vi "Value Change.vi"(8 "error in (no error)":errorcluster, 9 "NewVal":i32, 10 "Debugger":refnum<class "Debug Process.lvclass">, 11 "List Box View Model In":refnum<class "Multicolumn List Box View Model.lvclass">) -> (0 "error out":errorcluster, 3 "List Box View Model Out":refnum<class "Multicolumn List Box View Model.lvclass">)   [LabVIEW 2020, in "Multicolumn List Box View Model.lvclass"]
uses:
  Multicolumn List Box View Model.lvclass
  Process/Debug Process.lvclass
  Debugger/Debugger.lvclass
  Multicolumn List Box View Model.lvclass/Multicolumn List Box View Model.ctl
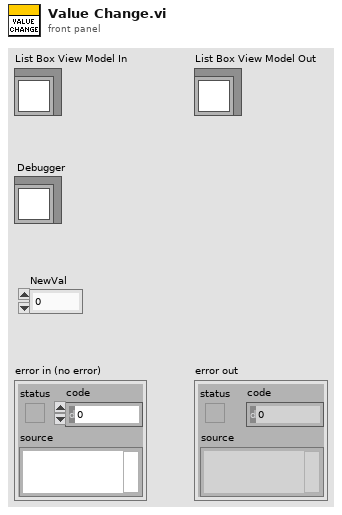
[diagram p1: front panel]
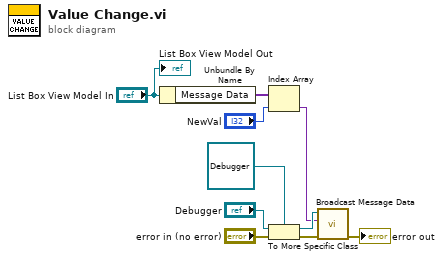
[diagram p0: block diagram]
diagram:
  n1 = Unbundle By Name("List Box View Model In") -> ("Message Data"=w4:variant[])
  n2 = Index Array(array=w4, index="NewVal") -> (element=w2:variant)
  n3 = To More Specific Class(target class=refnum<class "Debugger.lvclass"> refnum ("Debugger out"), reference="Debugger", error in="error in (no error)") -> (specific class reference=w9:refnum<class "Debugger.lvclass">, error out=w6:errorcluster)
  n4 = call "Broadcast Message Data.vi"("error in (no error)"=w6, "Message Data"=w2, "Debugger in"=w9) -> ("error out"=→"error out":errorcluster)  [unwired: 7 in, 1 out]
  "List Box View Model Out" <- "List Box View Model In"
